vi "Config.vi"(10 "Model Name":string, 11 "TaskConfig":refnum<data-value>) -> ()   [LabVIEW 2025, in "DAQ_Module.lvlib" / "DAQ_Module.lvclass"]
uses:
  DAQ_Module.lvclass
  DAQ_Config.ctl
  DAQ_Task_Config.ctl
  DAQ_HW_Type.ctl
  DAQ_Task_Type.ctl
  DAQ_SampleRateConfig.ctl
  <vilib>/addons/_JKI Toolkits/State Machine/_JKI_lib_State_Machine.llb/Select State(s)_err__jki_lib_state_machine.vi
  <vilib>/addons/_JKI Toolkits/State Machine/_JKI_lib_State_Machine.llb/Periodic Trigger__ogtk__JKI-SM__jki_lib_state_machine.vi
  DAQ_Module.lvclass/DAQ_Module.ctl
panel:
  in  "Listbox":string[](tree)
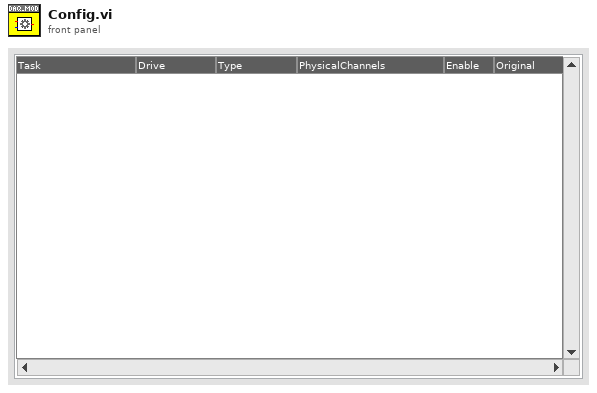
[diagram p1: front panel]
types:
  T1 = enum32{"Invalid", "Standard", "Closed", "Hidden", "Minimized", "Maximized"}
  T2 = enum32{"invalid app kind", "Development System", "Run Time System", "Student Edition", "Embedded LabVIEW", "Evaluation", "Custom"}
  T3 = typedef "LVPoint32TypeDef.ctl" = cluster{"Horizontal":i32, "Vertical":i32}
  T4 = typedef "DAQ_Module.lvlib/DAQ_Module.lvclass/DAQ_Config.ctl" = map{string, T5}
  T5 = typedef "DAQ_Module.lvlib/DAQ_Module.lvclass/DAQ_Task_Config.ctl" = cluster{"Drive":T6, "TaskType":T7, "PhysicalChannels":string, "SampleRateConfiguration":T8, "ChannelConfig":map{string, cluster{"Name":string, "Config":string}}, "Enable":bool, "Original":bool}
  T6 = typedef "DAQ_Module.lvlib/DAQ_Module.lvclass/DAQ_HW_Type.ctl" = enum16{"NI_DAQmx", "Simulated_DAQ"}
  T7 = typedef "DAQ_Module.lvlib/DAQ_Module.lvclass/DAQ_Task_Type.ctl" = enum16{"AI", "Linear", "Angular", "AO"}
  T8 = typedef "DAQ_Module.lvlib/DAQ_Module.lvclass/DAQ_SampleRateConfig.ctl" = cluster{"SampleRate":dbl, "SamplesPerChannel":u32, "SamplesPerRead":i32, "SampleMode":i32, "Clock Source":string}
  T9 = cluster{"Core":cluster{"Current VI Reference":refnum<vi>, "Close Panel on Exit?":bool}, "TaskConfig":refnum<data-value>, "Listbox":refnum<vi>, "Map":T4}
  T10 = cluster{"Current VI Reference":refnum<vi>, "Close Panel on Exit?":bool}
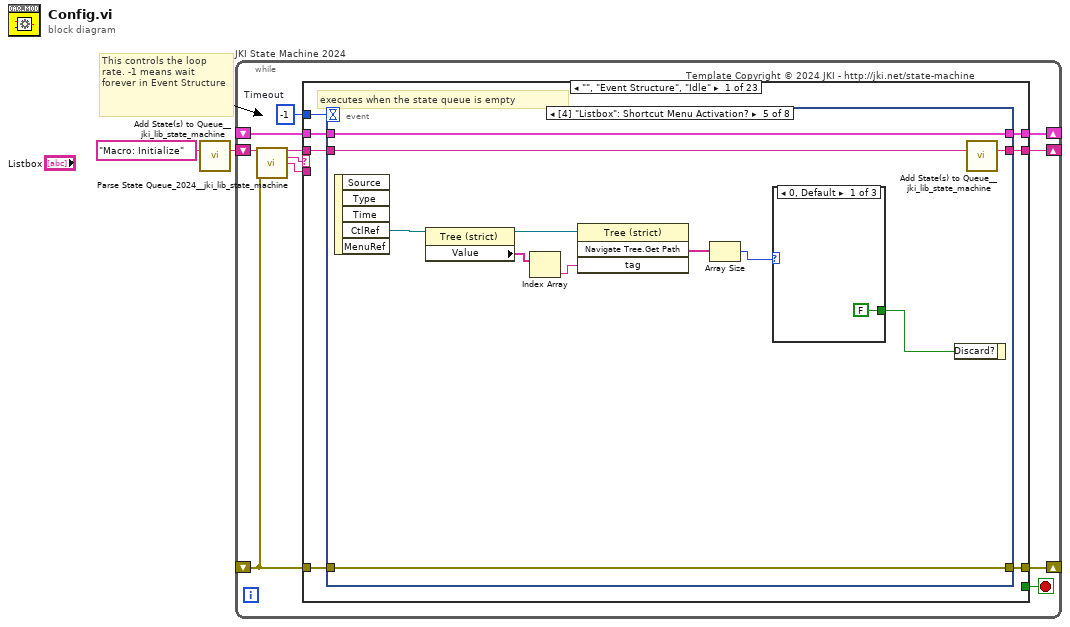
[diagram p0: block diagram]
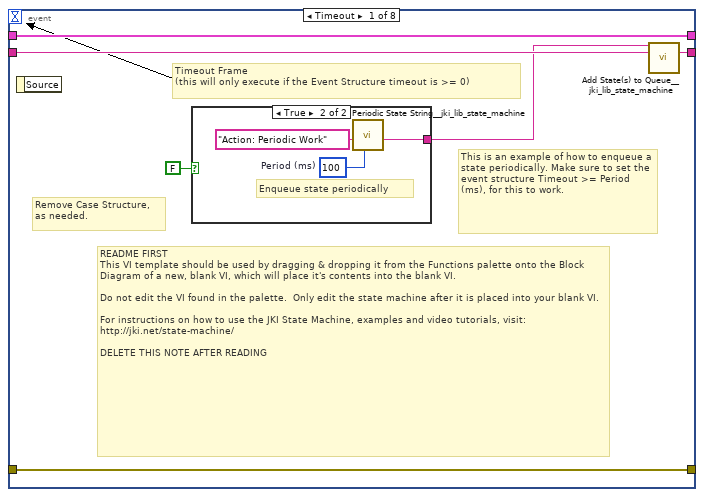
[diagram p2: hidden frame]
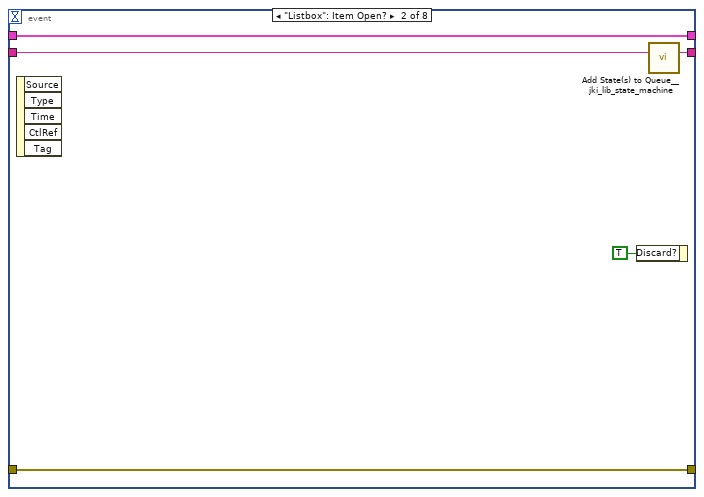
[diagram p4: hidden frame]
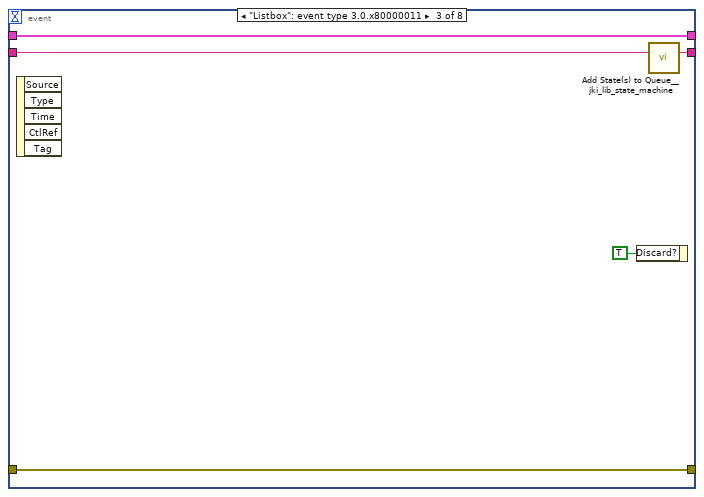
[diagram p5: hidden frame]
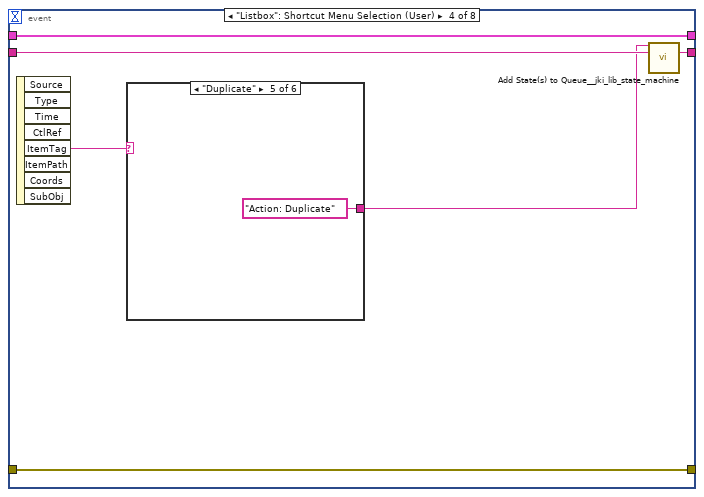
[diagram p6: hidden frame]
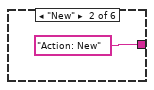
[diagram p8: hidden frame]
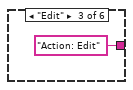
[diagram p9: hidden frame]
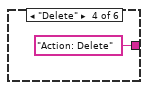
[diagram p10: hidden frame]
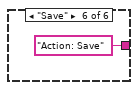
[diagram p11: hidden frame]
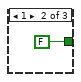
[diagram p12: hidden frame]
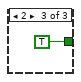
[diagram p13: hidden frame]
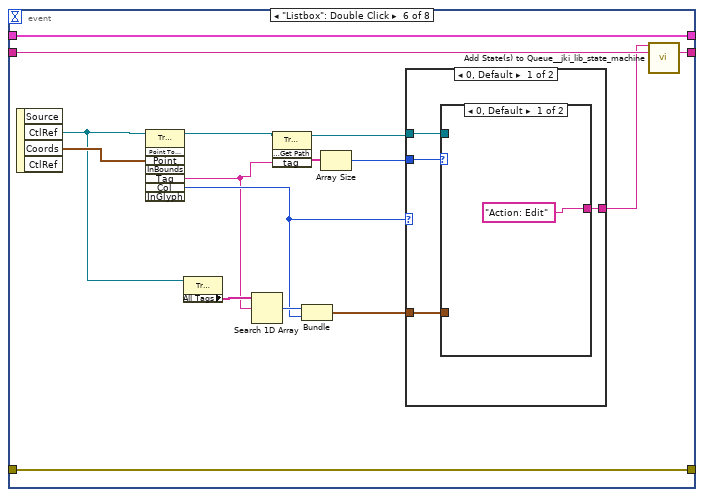
[diagram p14: hidden frame]
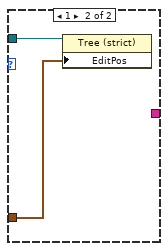
[diagram p15: hidden frame]
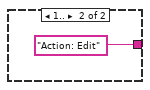
[diagram p16: hidden frame]
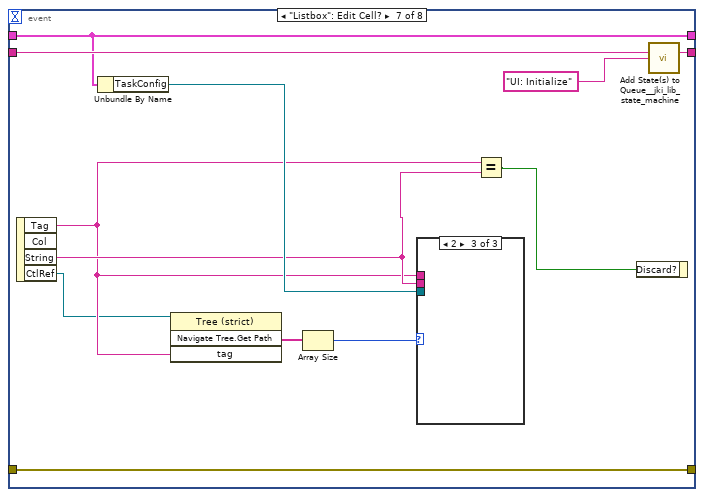
[diagram p17: hidden frame]
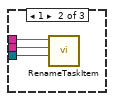
[diagram p19: hidden frame]
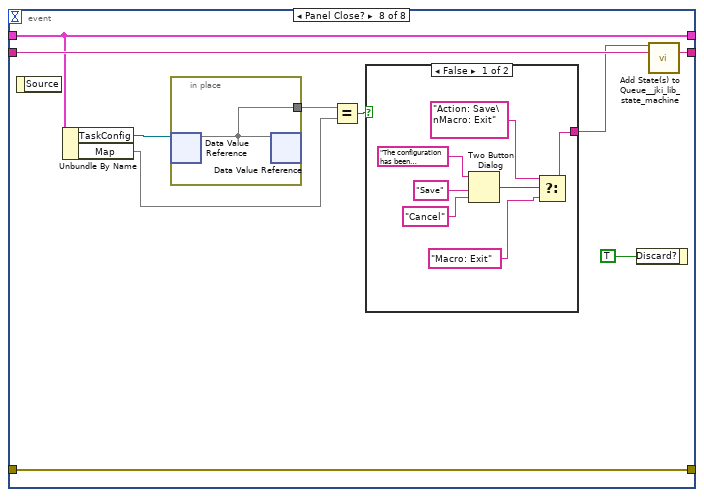
[diagram p20: hidden frame]
diagram:
  # "This controls the loop rate. -1 means wait forever in Event Structure"
  n1 = call <vilib>:"Add State(s) to Queue__jki_lib_state_machine.vi"("State(s) in (\"\")"="Macro: Initialize") -> ("States Out"=w2:string)  [unwired: 14 in]
  n2 = while "JKI State Machine 2024" {
    shift-right: [w6] -> _
    shift-left: _ -> [w5]
    shift-right: [w9] -> _
    shift-left: _ -> [w3]
    shift-right: [w8] -> _
    shift-left: w2 -> [w10]
    stop <- w7 stop-if-true
    w4 = -1  # Timeout
    # "Template Copyright © 2024 JKI - http://jki.net/state-machine"
    n3 = call <vilib>:"Parse State Queue_2024__jki_lib_state_machine.vi"("State Queue"=w10, "Error In (no error)"=w3) -> ("Remaining States"=w12:string, "Current State"=w13:string, "Arguments"=w11:string)  [unwired: 11 in]
    n4 = case shown="\"\", \"Event Structure\", \"Idle\"" w13 {
      selector: w13 -> [_ _ w127 _ _ _ _ _ _ _ _ _ _ _ _ _ _ _ _ _ _ _ _]
      tunnel: w12 -> [w20 w126 w131 w150 w160 w169 w173 w183 w190 w194 w201 w206 w212 w223 w292 w297 w306 w310 w316 w328 w341 w349 w359]
      tunnel: w11 -> [_ _ _ _ w155 _ _ _ _ _ _ _ w207 w217 _ _ _ _ _ _ _ _ _]
      tunnel: w5 -> [w18 w123 w129 w143 w157 w167 w170 _ w185 w191 w198 w204 w210 w219 w289 w294 w304 w307 w313 w325 w336 w345 w354]
      tunnel: [w17 w124 w133 w147 errorcluster {"status"=FALSE, "code"=0, "source"=""} ("error out") w166 w171 w180 w186 w192 w199 w203 w208 w220 w290 w295 w301 w308 w314 w326 w339 w347 w357] -> w9
      tunnel: w3 -> [w14 w124 w132 w147 w156 w166 w171 w180 w187 w192 w199 w203 w209 w221 w290 w295 w301 w308 w314 w326 w339 w347 w357]
      tunnel: [w19 w125 w130 w149 w159 w168 w172 w182 w189 w193 w200 w205 w211 w222 w291 w296 w305 w309 w315 w327 w340 w348 w358] -> w8
      tunnel: [_ _ _ _ _ TRUE _ _ _ _ _ _ _ _ _ _ _ _ _ _ _ _ _] -> w7
      tunnel: [w16 w123 w129 w148 w157 w167 w170 w181 w185 w191 w198 w204 w210 w219 w289 w294 w304 w307 w313 w325 w336 w345 w352] -> w6
      tunnel: w4 -> [w15 _ _ _ _ _ _ _ _ _ _ _ _ _ _ _ _ _ _ _ _ _ _]
      frame "", "Event Structure", "Idle" {
        # "executes when the state queue is empty"
        n5 = event shown="[4] \"Listbox\": Shortcut Menu Activation?" {
          selector: _ -> [_ _ _ _ _ _ _ _]
          dyn-events: _ -> [_ _ _ _ _ _ _ _]
          timeout: w15 -> [_ _ _ _ _ _ _ _]
          tunnel: w20 -> [w26 w34 w39 w45 w61 w80 w100 w113]
          tunnel: [w25 w33 w38 w44 w60 w79 w99 w112] -> w19
          tunnel: w18 -> [w23 w31 w36 w42 w58 w77 w97 w106]
          tunnel: [w24 w32 w37 w43 w59 w78 w98 w111] -> w17
          tunnel: w14 -> [w24 w32 w37 w43 w59 w78 w98 w111]
          tunnel: [w23 w31 w36 w42 w58 w77 w97 w106] -> w16
          event Timeout {
            # "Remove Case Structure, as needed."
            # "This is an example of how to enqueue a state periodically. Make sure to set the event structure Timeout >= Period (ms), for this to work."
            # "README FIRST\nThis VI template should be used by dragging & dropping it from the Functions palette onto the Block Diagram of a new, blank VI, which will place it's contents into the blank VI.\n\nDo not edit the VI found in the palette.  Only edit the state machine after it is placed into your blank VI.\n\nFor instructions on how to use the JKI State Machine, examples and video tutorials, visit:\nhttp://jki.net/state-machine/\n\nDELETE THIS NOTE AFTER READING"
            # "Timeout Frame\n(this will only execute if the Event Structure timeout is >= 0)"
            n6 = event-data() -> ()  [unwired: 1 in, 1 out]
            n7 = case shown="True" FALSE {
              tunnel: [_ w29] -> w22
              frame False {
              }
              frame True {
                w27 = u32 100  # Period (ms)
                # "Enqueue state periodically"
                n8 = call <vilib>:"Periodic State String__jki_lib_state_machine.vi"("Period (ms)"=w27, "State"="Action: Periodic Work") -> ("State Out"=w29:string)  [unwired: 9 in]
              }
            }
            n9 = call <vilib>:"Add State(s) to Queue__jki_lib_state_machine.vi"("State(s) in Front (\"\")"=w22, "State(s) in (\"\")"=w26) -> ("States Out"=w25:string)  [unwired: 13 in]
          }
          event "Listbox": Item Open? {
            n10 = event-data() -> ()  [unwired: 1 in, 5 out]
            n11 = event-data("Discard?"=TRUE) -> ()  [unwired: 1 in, 1 out]
            n12 = call <vilib>:"Add State(s) to Queue__jki_lib_state_machine.vi"("State(s) in (\"\")"=w34) -> ("States Out"=w33:string)  [unwired: 14 in]
          }
          event "Listbox": event type 3.0.x80000011 {
            n13 = event-data() -> ()  [unwired: 1 in, 5 out]
            n14 = event-data("Discard?"=TRUE) -> ()  [unwired: 1 in, 1 out]
            n15 = call <vilib>:"Add State(s) to Queue__jki_lib_state_machine.vi"("State(s) in (\"\")"=w39) -> ("States Out"=w38:string)  [unwired: 14 in]
          }
          event "Listbox": Shortcut Menu Selection (User) {
            n16 = event-data() -> ("ItemTag"=w41:string)  [unwired: 1 in, 7 out]
            n17 = case shown="\"Duplicate\"" w41 {
              tunnel: [_ "Action: New" "Action: Edit" "Action: Delete" "Action: Duplicate" "Action: Save"] -> w40
              frame Default {
              }
              frame "New" {
              }
              frame "Edit" {
              }
              frame "Delete" {
              }
              frame "Duplicate" {
              }
              frame "Save" {
              }
            }
            n18 = call <vilib>:"Add State(s) to Queue__jki_lib_state_machine.vi"("State(s) in Front (\"\")"=w40, "State(s) in (\"\")"=w45) -> ("States Out"=w44:string)  [unwired: 13 in]
          }
          event "Listbox": Shortcut Menu Activation? {
            n19 = event-data() -> ("CtlRef"=w56:refnum<vi>)  [unwired: 1 in, 4 out]
            n20 = property class="Tree (strict)"(reference=w56) -> (reference out=w55:refnum<vi>, "Value"=w54:string[])  [unwired: 1 in, 1 out]
            n21 = Index Array(array=w54) -> (element=w53:string)  [unwired: 1 in]
            n22 = invoke class="Tree (strict)" method="Navigate Tree.Get Path"(reference=w55, "tag"=w53) -> ("Navigate Tree:Get Path"=w57:string[])  [unwired: 2 in, 3 out]
            n23 = Array Size(array=w57) -> (size(s)=w52:i32)
            n24 = case shown="0, Default" w52 {
              tunnel: [FALSE FALSE TRUE] -> w51
              frame 0, Default {
              }
              frame 1 {
              }
              frame 2 {
              }
            }
            n25 = event-data("Discard?"=w51) -> ()  [unwired: 1 in, 1 out]
            n26 = call <vilib>:"Add State(s) to Queue__jki_lib_state_machine.vi"("State(s) in (\"\")"=w61) -> ("States Out"=w60:string)  [unwired: 14 in]
          }
          event "Listbox": Double Click {
            n27 = event-data() -> ("CtlRef"=w74:refnum<vi>, "Coords"=w75:T3)  [unwired: 1 in, 2 out]
            n28 = invoke class="Tree (strict)" method="Point To Row Column"(reference=w74, "Point"=w75) -> (reference out=w68:refnum<vi>, "Tag"=w66:string, "Col"=w71:i32)  [unwired: 6 in, 5 out]
            n29 = property class="Tree (strict)"(reference=w74) -> ("All Tags"=w73:string[])  [unwired: 1 in, 2 out]
            n30 = Search 1D Array(1D array=w73, element=w66) -> (index of element=w72:i32)  [unwired: 1 in]
            n31 = invoke class="Tree (strict)" method="Navigate Tree.Get Path"(reference=w68, "tag"=w66) -> (reference out=w67:refnum<vi>, "Navigate Tree:Get Path"=w69:string[])  [unwired: 2 in, 2 out]
            n32 = Bundle("index of element"=w72, "Col"=w71) -> (w70:cluster{"index of element":i32, "Col":i32})  [unwired: 1 in]
            n33 = Array Size(array=w69) -> (size(s)=w65:i32)
            n34 = case shown="0, Default" w71 {
              tunnel: [w81 "Action: Edit"] -> w76
              tunnel: w67 -> [w84 _]
              tunnel: w70 -> [w83 _]
              tunnel: w65 -> [w82 _]
              frame 0, Default {
                n35 = case shown="0, Default" w82 {
                  tunnel: w84 -> [_ w87]
                  tunnel: w83 -> [_ w86]
                  tunnel: ["Action: Edit" _] -> w81
                  frame 0, Default {
                  }
                  frame 1 {
                    n36 = property class="Tree (strict)"(reference=w87, "EditPos"=w86) -> ()  [unwired: 1 in, 2 out]
                  }
                }
              }
              frame 1.. {
              }
            }
            n37 = call <vilib>:"Add State(s) to Queue__jki_lib_state_machine.vi"("State(s) in Front (\"\")"=w76, "State(s) in (\"\")"=w80) -> ("States Out"=w79:string)  [unwired: 13 in]
          }
          event "Listbox": Edit Cell? {
            n38 = event-data() -> ("Tag"=w91:string, "String"=w93:string, "CtlRef"=w90:refnum<vi>)  [unwired: 1 in, 1 out]
            n39 = Unbundle By Name(w97) -> ("TaskConfig"=w96:refnum<data-value>)
            n40 = invoke class="Tree (strict)" method="Navigate Tree.Get Path"(reference=w90, "tag"=w91) -> ("Navigate Tree:Get Path"=w92:string[])  [unwired: 2 in, 3 out]
            n41 = Array Size(array=w92) -> (size(s)=w89:i32)
            n42 = case shown="2" w89 {
              tunnel: w96 -> [_ w103 _]
              tunnel: w93 -> [_ w102 _]
              tunnel: w91 -> [_ w101 _]
              frame 0, Default {
              }
              frame 1 {
                n43 = call "RenameTaskItem.vi"("TaskConfig"=w103, "New Task"=w102, "Old Task"=w101) -> ()  [unwired: 9 in]
              }
              frame 2 {
              }
            }
            n44 = Equal?(x=w91, y=w93) -> (x = y?=w95:bool)
            n45 = event-data("Discard?"=w95) -> ()  [unwired: 1 in, 1 out]
            n46 = call <vilib>:"Add State(s) to Queue__jki_lib_state_machine.vi"("State(s) in (\"\")"=w100, "State(s) at Back (\"\")"="UI: Initialize" ("State(s) at Back (\"\")")) -> ("States Out"=w99:string)  [unwired: 13 in]
          }
          event Panel Close? {
            n47 = event-data() -> ()  [unwired: 1 in, 1 out]
            n48 = Unbundle By Name(w106) -> ("TaskConfig"=w109:refnum<data-value>, "Map"=w108:T4)
            n49 = in-place {
              in-place-border: [w122] -> w107
              n50 = in-place-dvr #1(w109) -> (w122:T4)  [unwired: 1 out]
              n51 = in-place-dvr #1(w122) -> ()  [unwired: 2 out]
            }
            n52 = Equal?(x=w107, y=w108) -> (x = y?=w105:bool)
            n53 = case shown="False" w105 {
              tunnel: [w115 "Macro: Exit"] -> w104
              frame False {
                n54 = Two Button Dialog(message="The configuration has been modified. \nDo you wish to save the changes?", 1:"Cancel" ("F button name (\"Cancel\")"), 2:"Save" ("T button name (\"OK\")")) -> (T button?=w117:bool)
                n55 = Select(t="Action: Save\nMacro: Exit", s=w117, f="Macro: Exit") -> (s? t:f=w115:string)
              }
              frame True {
              }
            }
            n56 = event-data("Discard?"=TRUE) -> ()  [unwired: 1 in, 1 out]
            n57 = call <vilib>:"Add State(s) to Queue__jki_lib_state_machine.vi"("State(s) in Front (\"\")"=w104, "State(s) in (\"\")"=w113) -> ("States Out"=w112:string)  [unwired: 13 in]
          }
        }
      }
      frame "---------- Core ----------" {
        # "Do not put any code in this frame.\n(it is a separator no-op)"
        n58 = call <vilib>:"Add State(s) to Queue__jki_lib_state_machine.vi"("State(s) in (\"\")"=w126) -> ("States Out"=w125:string)  [unwired: 14 in]
      }
      frame Default {
        w136 = 42 items=["No error", "Argument error", "Memory is full", "Out of zone", "End of file", "File already open", "Generic file I/O error", "File not found", "File permission error", "Disk is full", "Duplicate path", "Too many files open", "System feature not enabled", "Resource file not found", "Cannot add resource", "Resource not found", "Image not found", "Image memory error", "Pen does not exist", "Config type invalid", "Config token not found", "Config parse error", "Config memory error", "Bad external code format", "Bad external code offset", "External code not present", "Null window", "Destroy window error", "Null menu", "Print aborted", "Bad print record", "Print driver error", "Windows error during printing", "Memory error during printing", "Print dialog error", "Generic print error", "Invalid device refnum", "Device not found", "Device parameter error", "Device unit error", "Cannot open device", "Device call aborted", "Generic error", "Cancelled by user", "Object ID too low", "Object ID too high", "Object not in heap", "Unknown heap", "Unknown object (invalid DefProc)", "Unknown object (DefProc not in table)", "Message out of range", "Invalid (null) method", "Unknown message", "Manager call not supported", "Bad address", "Network operation in progress", "Network operation timed out", "Connection is busy", "Network attribute not supported", "Network error", "Address in use", "System out of memory", "Connection aborted", "Connection refused", "Not connected", "Already connected", "Connection closed", "Initialization error (interapplication manager)", "Bad occurrence", "Wait on unbound occurrence handler", "Occurrence queue overflow", "Datalog type conflict", "Unused", "Unrecognized type (interapplication manager)", "Memory corrupt", "Failed to make temporary DLL", "Old CIN version", "Drag socket not found", "Failed to load drop-object", "Failed to register OLE object", "Failed to release OLE object", "Format specifier type mismatch", "Unknown format specifier", "Too few format specifiers", "Too many format specifiers", "Scan failed", "Newer CIN version", "Error converting to variant", "Runtime menu error", "Password tampered", "Variant attribute not found", "Incompatible variant data type", "Event data is not available", "Event Store is not present", "Occurrence is not found", "Event Queue is not created", "Event info is not available", "Refnum passed is NULL", "Error retrieving Class GUID", "Error retrieving CoClass GUID", "Error retrieving TypeLib GUID.", "Bad built application magic bytes.", "Specific driver is different from the specific driver associated with the Logical Name.", "There is no session opened to the class driver.", "Max Error", "MAX - Error with config objects", "MAX - Error loading configuration", "MAX - Group not supported"]
        # "Current State"
        # "Do not delete, rename, or modify this frame.\n(this is used to capture unhandled states and typos)"
        # "Handle mistyped state name (developer tool)"
        n59 = Format Into String(format string="Software Exception: Unhandled State \"%s\"." ("message"), error in=w132, w127) -> (resulting string=w135:string, error out=w134:errorcluster)  [unwired: 1 in]
        n60 = call <vilib>:"Error Cluster From Error Code.vi"("show call chain? (False)"=TRUE, "error in (no error)"=w134, "error message (\"\")"=w135, "error code (0)"=w136) -> ("error out"=w133:errorcluster)  [unwired: 5 in]
        n61 = call <vilib>:"Add State(s) to Queue__jki_lib_state_machine.vi"("State(s) in (\"\")"=w131) -> ("States Out"=w130:string)  [unwired: 14 in]
      }
      frame "Initialize Core Data" {
        # "Do not delete, rename, or modify this frame.\n(this is used to determine panel behavior on exit)"
        # "originally closed?"
        # "exe?"
        # "If panel starts closed or is an EXE, then close it when we exit"
        n62 = property class="VI"() -> ("FP.State"=w140:T1)  [unwired: 2 in, 2 out]
        n63 = property class="App"() -> ("App.Kind"=w146:T2)  [unwired: 2 in, 2 out]
        n64 = control-ref of="Current VI Reference"() -> (w141:refnum<vi>)
        n65 = Equal?(x=w140, y=T1."Closed" ("Front Panel Window:State")) -> (x = y?=w138:bool)
        n66 = Equal?(x=w146, y=T2."Run Time System" ("Application:Kind")) -> (x = y?=w144:bool)
        n67 = Or(x=w138, y=w144) -> (x .or. y?=w142:bool)
        n68 = Bundle By Name(cluster=w143, "Core.Current VI Reference"=w141, "Core.Close Panel on Exit?"=w142) -> (w148:T9)
        n69 = call <vilib>:"Add State(s) to Queue__jki_lib_state_machine.vi"("State(s) in (\"\")"=w150) -> ("States Out"=w149:string)  [unwired: 14 in]
      }
      frame "Error Handler" {
        # "When running as sourcecode, this function will add previous state data to the error message to aid the developer in troubleshoot errors.\nIf run as an executable, no additional information is added to the error message."
        # "This state receives both Errors and Warnings which is how the Status of this wire can be FALSE"
        # "Unhandled Error -- Display it"
        # "Handle any errors or warnings here.\nYou can also output any states to clean-up after errors or warnings occur"
        # "Clear error or warning"
        n70 = disable-structure shown="Default" {
          disable-tunnel: w156 -> [w163 w164]
          disable-tunnel: w155 -> [w162 _]
          disable-tunnel: [w161 w164] -> w154
          frame condition #0 (active) {
            n71 = call <vilib>:"Append Error Details__jki_lib_state_machine.vi"("error in (no error)"=w163, "Previous State and Argument(s)"=w162) -> ("error out"=w161:errorcluster)  [unwired: 9 in]
          }
          frame condition #1 {
          }
        }
        n72 = call <vilib>:"General Error Handler.vi"("error in (no error)"=w154) -> ()  [unwired: 10 in, 5 out]
        n73 = call-poly <vilib>:"Select State(s)__jki_lib_state_machine.vi"("State(s) if True (\"\")"="/* Post Error States", "Select"=w154, "State(s) if False (\"\")"="/* Post Warning States") -> ("States Out"=w152:string)  [unwired: 12 in]
        n74 = call <vilib>:"Add State(s) to Queue__jki_lib_state_machine.vi"("State(s) in Front (\"\")"=w152, "State(s) in (\"\")"=w160) -> ("States Out"=w159:string)  [unwired: 13 in]
      }
      frame "Exit" {
        # "Do not put any code in this frame.\n(No errors that occur here will be handled.)"
        n75 = call <vilib>:"Add State(s) to Queue__jki_lib_state_machine.vi"("State(s) in (\"\")"=w169) -> ("States Out"=w168:string)  [unwired: 14 in]
      }
      frame "---------- Data ----------" {
        # "Do not put any code in this frame.\n(It is a separator no-op. You can make a copy of this frame to create a new Data frame)"
        n76 = call <vilib>:"Add State(s) to Queue__jki_lib_state_machine.vi"("State(s) in (\"\")"=w173) -> ("States Out"=w172:string)  [unwired: 14 in]
      }
      frame "Data: Initialize" {
        w179 = T10 {"Current VI Reference"=refnum, "Close Panel on Exit?"=FALSE}  # Core
        # "Data names and types of shift register data are defined by this bundle."
        # "Initialize the shift-register data, here.\n(data names are defined by what you wire into the bundle function)"
        n77 = control-ref of="Listbox"() -> (w178:refnum<vi>)
        n78 = property class="Tree (strict)"(reference=w178, "AlternatingRowColors"=TRUE ("Alternating Row Colors")) -> (reference out=w175:refnum<vi>)  [unwired: 1 in, 1 out]
        n79 = in-place {
          in-place-border: [w184] -> w176
          n80 = in-place-dvr #2("TaskConfig") -> (w184:T4)  [unwired: 1 out]
          n81 = in-place-dvr #2(w184) -> ()  [unwired: 2 out]
        }
        n82 = Bundle("Core"=w179, "TaskConfig"="TaskConfig", "Listbox"=w175, "Map"=w176) -> (w181:T9)  [unwired: 1 in]
        n83 = call <vilib>:"Add State(s) to Queue__jki_lib_state_machine.vi"("State(s) in (\"\")"=w183) -> ("States Out"=w182:string)  [unwired: 14 in]
      }
      frame "Data: Cleanup" {
        # "Cleanup any data and references, here.\n(this is called automatically, by the Macro: Exit)"
        n84 = Unbundle By Name(w185) -> ("Core.Current VI Reference"=w188:refnum<vi>)
        n85 = Close Reference(reference=w188, error in (no error)=w187) -> (error out=w186:errorcluster)
        n86 = call <vilib>:"Add State(s) to Queue__jki_lib_state_machine.vi"("State(s) in (\"\")"=w190) -> ("States Out"=w189:string)  [unwired: 14 in]
      }
      frame "---------- UI ----------" {
        # "Do not put any code in this frame.\n(It is a separator no-op. You can make a copy of this frame to create a new UI frame)"
        n87 = call <vilib>:"Add State(s) to Queue__jki_lib_state_machine.vi"("State(s) in (\"\")"=w194) -> ("States Out"=w193:string)  [unwired: 14 in]
      }
      frame "UI: Initialize" {
        # "Initialize the User Interface, here.\n(this is called automatically, by the Macro: Initialize)"
        n88 = Unbundle By Name(w198) -> ("Listbox"=w195:refnum<vi>, "TaskConfig"=w197:refnum<data-value>)
        n89 = in-place {
          in-place-border: [w202] -> w196
          n90 = in-place-dvr #3(w197) -> (w202:T4)  [unwired: 1 out]
          n91 = in-place-dvr #3(w202) -> ()  [unwired: 2 out]
        }
        n92 = call "UI(Edit_Init).vi"("Map"=w196, "Listbox"=w195) -> ()  [unwired: 10 in]
        n93 = call <vilib>:"Add State(s) to Queue__jki_lib_state_machine.vi"("State(s) in (\"\")"=w201) -> ("States Out"=w200:string)  [unwired: 14 in]
      }
      frame "UI: Uninitialize" {
        # "Cleanup the User Interface, here.\n(this is called automatically, by the Macro: Exit)"
        n94 = call <vilib>:"Add State(s) to Queue__jki_lib_state_machine.vi"("State(s) in (\"\")"=w206) -> ("States Out"=w205:string)  [unwired: 14 in]
      }
      frame "UI: Cursor Set" {
        # "Argument"
        # "Set and Unset Cursor Busy.\n(Usage: \"UI: Cursor Set >> Busy|Idle\")"
        n95 = case shown="\"Idle\", Default" w207 {
          tunnel: w209 -> [w214 w216]
          tunnel: [w213 w215] -> w208
          frame "Idle", Default {
            n96 = call <vilib>:"Unset Busy.vi"("error in (no error)"=w214) -> ("error out"=w213:errorcluster)  [unwired: 10 in]
          }
          frame "Busy" {
            n97 = call <vilib>:"Set Busy.vi"("error in (no error)"=w216) -> ("error out"=w215:errorcluster)  [unwired: 9 in, 1 out]
          }
        }
        n98 = call <vilib>:"Add State(s) to Queue__jki_lib_state_machine.vi"("State(s) in (\"\")"=w212) -> ("States Out"=w211:string)  [unwired: 14 in]
      }
      frame "UI: Front Panel State" {
        # "Argument"
        # "Set Front Panel Open or Closed\n(Usage: \"UI: Front Panel State >> Open|Close\")"
        n99 = Unbundle By Name(w219) -> ("Core.Current VI Reference"=w218:refnum<vi>)
        n100 = case shown="\"Minimize\", \"Minimized\"" w217 {
          tunnel: w221 -> [w229 w244 w255 w268 w281]
          tunnel: [w231 w245 w257 w270 w283] -> w220
          tunnel: w218 -> [w230 w242 w256 w269 w282]
          frame "Open", "Standard", Default {
            w224 = T1."Standard" ("State")
            n101 = property class="VI"(reference=w230, error in=w229) -> (reference out=w227:refnum<vi>, error out=w228:errorcluster, "FP.State"=w226:T1)
            n102 = Not Equal?(x=w226, y=w224) -> (x != y?=w225:bool)
            n103 = case shown="True" w225 {
              tunnel: [w235 w237] -> w231
              tunnel: w228 -> [w234 w237]
              tunnel: w227 -> [w233 _]
              tunnel: w224 -> [w232 _]
              frame True {
                n104 = invoke class="VI" method="FP.Open"(reference=w233, error in=w234, "Activate"=TRUE, "State"=w232) -> (error out=w235:errorcluster)  [unwired: 1 in, 4 out]
              }
              frame False {
              }
            }
          }
          frame "Close", "Closed" {
            n105 = property class="VI"(reference=w242, error in=w244) -> (reference out=w241:refnum<vi>, error out=w243:errorcluster, "FP.State"=w239:T1)
            n106 = Not Equal?(x=w239, y=T1."Closed" ("Front Panel Window:State")) -> (x != y?=w238:bool)
            n107 = case shown="True" w238 {
              tunnel: [w246 w249] -> w245
              tunnel: w243 -> [w246 w248]
              tunnel: w241 -> [_ w247]
              frame False {
              }
              frame True {
                n108 = invoke class="VI" method="FP.Close"(reference=w247, error in=w248) -> (error out=w249:errorcluster)  [unwired: 1 in, 2 out]
              }
            }
          }
          frame "Hidden", "Hide" {
            w250 = T1."Hidden" ("State")
            n109 = property class="VI"(reference=w256, error in=w255) -> (reference out=w253:refnum<vi>, error out=w254:errorcluster, "FP.State"=w252:T1)
            n110 = Not Equal?(x=w252, y=w250) -> (x != y?=w251:bool)
            n111 = case shown="True" w251 {
              tunnel: [w261 w262] -> w257
              tunnel: w254 -> [w260 w262]
              tunnel: w253 -> [w259 _]
              tunnel: w250 -> [w258 _]
              frame True {
                n112 = invoke class="VI" method="FP.Open"(reference=w259, error in=w260, "State"=w258) -> (error out=w261:errorcluster)  [unwired: 2 in, 4 out]
              }
              frame False {
              }
            }
          }
          frame "Minimize", "Minimized" {
            w263 = T1."Minimized" ("State")
            n113 = property class="VI"(reference=w269, error in=w268) -> (reference out=w266:refnum<vi>, error out=w267:errorcluster, "FP.State"=w265:T1)
            n114 = Not Equal?(x=w265, y=w263) -> (x != y?=w264:bool)
            n115 = case shown="True" w264 {
              tunnel: [w274 w275] -> w270
              tunnel: w267 -> [w273 w275]
              tunnel: w266 -> [w272 _]
              tunnel: w263 -> [w271 _]
              frame True {
                n116 = invoke class="VI" method="FP.Open"(reference=w272, error in=w273, "State"=w271) -> (error out=w274:errorcluster)  [unwired: 2 in, 4 out]
              }
              frame False {
              }
            }
          }
          frame "Maximize", "Maximized" {
            w276 = T1."Maximized" ("State")
            n117 = property class="VI"(reference=w282, error in=w281) -> (reference out=w279:refnum<vi>, error out=w280:errorcluster, "FP.State"=w278:T1)
            n118 = Not Equal?(x=w278, y=w276) -> (x != y?=w277:bool)
            n119 = case shown="True" w277 {
              tunnel: [w287 w288] -> w283
              tunnel: w280 -> [w286 w288]
              tunnel: w279 -> [w285 _]
              tunnel: w276 -> [w284 _]
              frame True {
                n120 = invoke class="VI" method="FP.Open"(reference=w285, error in=w286, "State"=w284) -> (error out=w287:errorcluster)  [unwired: 2 in, 4 out]
              }
              frame False {
              }
            }
          }
        }
        n121 = call <vilib>:"Add State(s) to Queue__jki_lib_state_machine.vi"("State(s) in (\"\")"=w223) -> ("States Out"=w222:string)  [unwired: 14 in]
      }
      frame "---------- Macro ----------" {
        # "Do not put any code in this frame.\n(It is a separator no-op. You can make a copy of this frame to create a new Macro frame)"
        n122 = call <vilib>:"Add State(s) to Queue__jki_lib_state_machine.vi"("State(s) in (\"\")"=w292) -> ("States Out"=w291:string)  [unwired: 14 in]
      }
      frame "Macro: Initialize" {
        w293 = "Data: Initialize\nInitialize Core Data\nUI: Initialize\nUI: Front Panel State >> Open"  # Data: Initialize Initialize Core Data UI: Initialize UI: Front Panel State >> Open
        # "Initialization Macro\n(This is called once, when the VI starts)"
        n123 = call <vilib>:"Add State(s) to Queue__jki_lib_state_machine.vi"("State(s) in Front (\"\")"=w293, "State(s) in (\"\")"=w297) -> ("States Out"=w296:string)  [unwired: 13 in]
      }
      frame "Macro: Exit" {
        # "Exit Macro\n(This is called once, when the VI exits)"
        n124 = Unbundle By Name(w304) -> ("Core.Close Panel on Exit?"=w299:bool)
        n125 = call <vilib>:"Conditional State String__jki_lib_state_machine.vi"("Do State(s)?"=w299, "State"="UI: Front Panel State >> Close") -> ("State Out"=w298:string)  [unwired: 7 in]
        n126 = call <vilib>:"Add State(s) to Queue__jki_lib_state_machine.vi"("State(s) in (\"\")"=w298, "State(s) at Back (\"\")"="UI: Uninitialize\nData: Cleanup\nExit") -> ("States Out"=w302:string)  [unwired: 13 in]
        n127 = call <vilib>:"Add State(s) to Queue__jki_lib_state_machine.vi"("State(s) in Front (\"\")"=w302, "State(s) in (\"\")"=w306) -> ("States Out"=w305:string)  [unwired: 13 in]
      }
      frame "---------- Action ----------" {
        # "Template Separator\n(You can make a copy of, or modify, this frame)"
        n128 = call <vilib>:"Add State(s) to Queue__jki_lib_state_machine.vi"("State(s) in (\"\")"=w310) -> ("States Out"=w309:string)  [unwired: 14 in]
      }
      frame "Action: New" {
        # "Your code here.\n(You can make a copy of, or modify, this frame)"
        n129 = Unbundle By Name(w313) -> ("TaskConfig"=w312:refnum<data-value>)
        n130 = call "NewTaskItem.vi"("TaskConfig"=w312) -> ()  [unwired: 11 in]
        n131 = call <vilib>:"Add State(s) to Queue__jki_lib_state_machine.vi"("State(s) in (\"\")"=w316, "State(s) at Back (\"\")"="UI: Initialize" ("State(s) at Back (\"\")")) -> ("States Out"=w315:string)  [unwired: 13 in]
      }
      frame "Action: Edit" {
        # "Your code here.\n(You can make a copy of, or modify, this frame)"
        n132 = Unbundle By Name(w325) -> ("Listbox"=w324:refnum<vi>, "TaskConfig"=w323:refnum<data-value>)
        n133 = property class="Tree (strict)"(reference=w324) -> (reference out=w320:refnum<vi>, "Value"=w321:string[])  [unwired: 1 in, 1 out]
        n134 = Index Array(array=w321) -> (element=w319:string)  [unwired: 1 in]
        n135 = invoke class="Tree (strict)" method="Navigate Tree.Get Path"(reference=w320, "tag"=w319) -> ("Navigate Tree:Get Path"=w318:string[])  [unwired: 2 in, 3 out]
        n136 = Array Size(array=w318) -> (size(s)=w317:i32)
        n137 = case shown="1" w317 {
          tunnel: w323 -> [_ w330 w331]
          tunnel: w319 -> [_ w329 w332]
          frame 0, Default {
          }
          frame 1 {
            n138 = call "Edit.vi"("TaskConfig"=w330, "TaskName"=w329) -> ()  [unwired: 10 in]
          }
          frame 2 {
            n139 = call "Edit(Channel).vi"("TaskConfig"=w331, "Tag"=w332) -> ()  [unwired: 10 in]
          }
        }
        n140 = call <vilib>:"Add State(s) to Queue__jki_lib_state_machine.vi"("State(s) in (\"\")"=w328, "State(s) at Back (\"\")"="UI: Initialize" ("State(s) at Back (\"\")")) -> ("States Out"=w327:string)  [unwired: 13 in]
      }
      frame "Action: Duplicate" {
        # "Your code here.\n(You can make a copy of, or modify, this frame)"
        n141 = Unbundle By Name(w336) -> ("Listbox"=w338:refnum<vi>, "TaskConfig"=w335:refnum<data-value>)
        n142 = property class="Tree (strict)"(reference=w338) -> ("Value"=w337:string[])  [unwired: 1 in, 2 out]
        n143 = Index Array(array=w337) -> (element=w333:string)  [unwired: 1 in]
        n144 = call "DuplicateTaskItem.vi"("TaskConfig"=w335, "Task"=w333) -> ()  [unwired: 10 in]
        n145 = call <vilib>:"Add State(s) to Queue__jki_lib_state_machine.vi"("State(s) in (\"\")"=w341, "State(s) at Back (\"\")"="UI: Initialize" ("State(s) at Back (\"\")")) -> ("States Out"=w340:string)  [unwired: 13 in]
      }
      frame "Action: Delete" {
        # "Your code here.\n(You can make a copy of, or modify, this frame)"
        n146 = Unbundle By Name(w345) -> ("Listbox"=w346:refnum<vi>, "TaskConfig"=w343:refnum<data-value>)
        n147 = property class="Tree (strict)"(reference=w346) -> ("Value"=w344:string[])  [unwired: 1 in, 2 out]
        n148 = for {
          tunnel: w344 -> [w350] mode=indexing
          tunnel: w343 -> [w351]
          n149 = call "DeleteTaskItem.vi"("TaskConfig"=w351, "Task"=w350) -> ()  [unwired: 10 in]
        }
        n150 = call <vilib>:"Add State(s) to Queue__jki_lib_state_machine.vi"("State(s) in (\"\")"=w349, "State(s) at Back (\"\")"="UI: Initialize" ("State(s) at Back (\"\")")) -> ("States Out"=w348:string)  [unwired: 13 in]
      }
      frame "Action: Save" {
        # "Template Separator\n(You can make a copy of, or modify, this frame)"
        n151 = Unbundle By Name(w354) -> ("TaskConfig"=w356:refnum<data-value>)
        n152 = in-place {
          in-place-border: [w360] -> w353
          n153 = in-place-dvr #4(w356) -> (w360:T4)  [unwired: 1 out]
          n154 = in-place-dvr #4(w360) -> ()  [unwired: 2 out]
        }
        n155 = call "SaveConfigFile.vi"("Map"=w353, "Model Name"="Model Name") -> ()  [unwired: 9 in, 1 out]
        n156 = Bundle By Name(cluster=w354, "Map"=w353) -> (w352:T9)
        n157 = call <vilib>:"Add State(s) to Queue__jki_lib_state_machine.vi"("State(s) in (\"\")"=w359) -> ("States Out"=w358:string)  [unwired: 14 in]
      }
    }
  }
